vi "Get Info.vi"(8 "error in (no error)":errorcluster, 11 "Category in":refnum<class "Category.lvclass">) -> (0 "error out":errorcluster, 1 "Name":string, 2 "id":i32, 3 "Category out":refnum<class "Category.lvclass">)   [LabVIEW 2018, in "Category.lvclass"]
uses:
  Category.lvclass
  Category.lvclass/Category.ctl
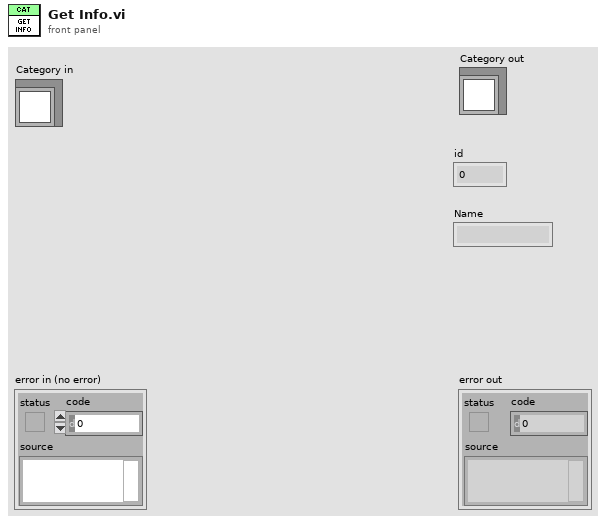
[diagram p1: front panel]
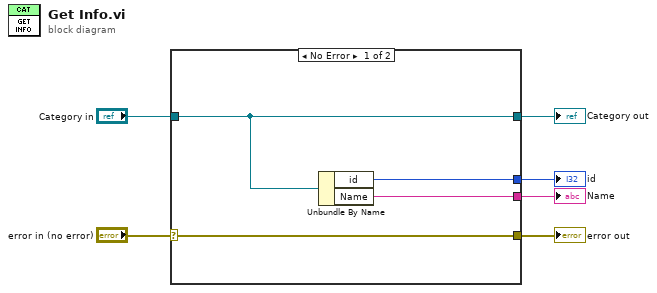
[diagram p0: block diagram]
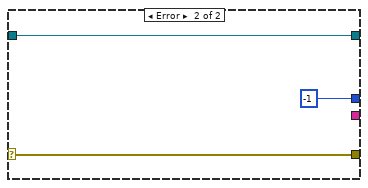
[diagram p2: hidden frame]
diagram:
  n1 = case shown="No Error" "error in (no error)" {
    selector: "error in (no error)" -> [w10 w13]
    tunnel: [w10 w13] -> w5
    tunnel: "Category in" -> [w7 w11]
    tunnel: [w9 _] -> w3
    tunnel: [w8 -1 ("id")] -> w2
    tunnel: [w7 w11] -> w1
    frame No Error {
      n2 = Unbundle By Name(w7) -> ("id"=w8:i32, "Name"=w9:string)
    }
    frame Error {
    }
  }
  "error out" <- w5
  "Name" <- w3
  "id" <- w2
  "Category out" <- w1
